vi "Primitives.vi"(1 "Angle to Target":i32, 5 "Primitive":string, 8 "Distance to Target":i32) -> (0 "Port Speed":i32, 6 "Starboard Speed":i32)   [LabVIEW 2012]
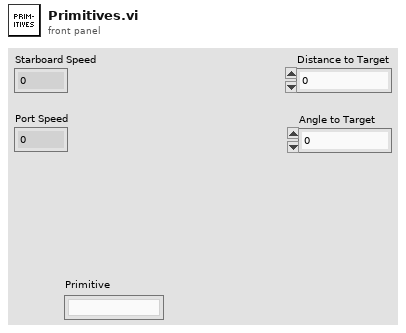
[diagram p1: front panel]
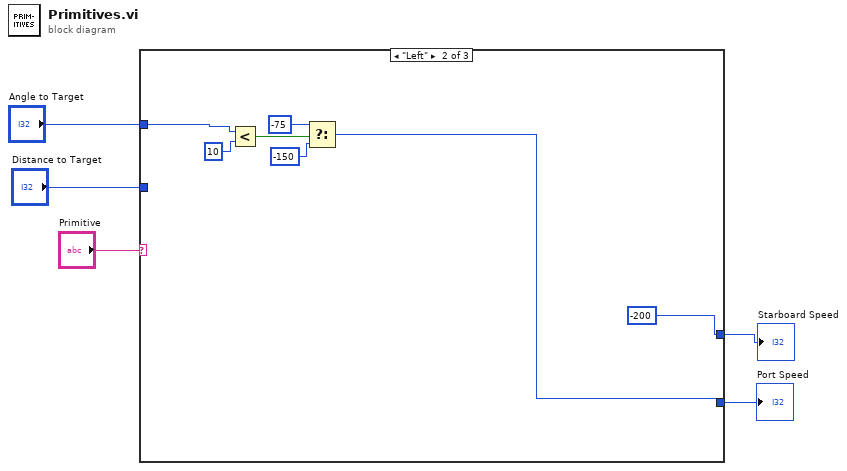
[diagram p0: block diagram]
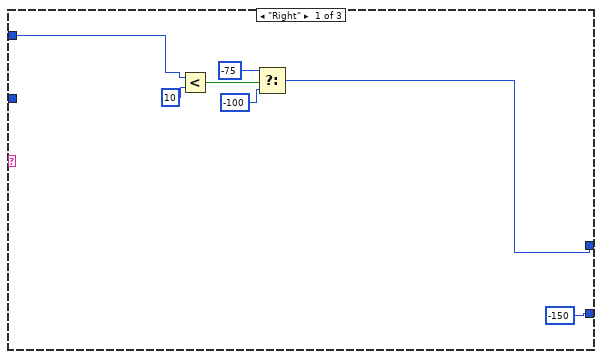
[diagram p2: hidden frame]
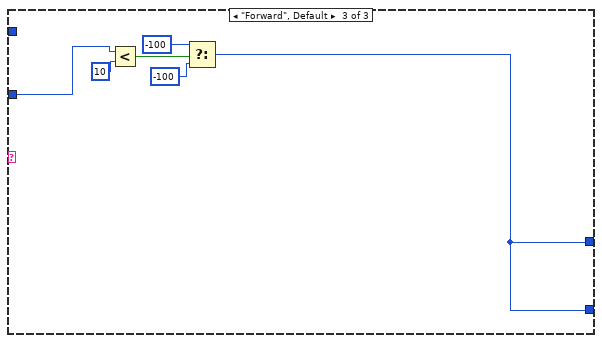
[diagram p3: hidden frame]
diagram:
  n1 = case shown="\"Left\"" "Primitive" {
    tunnel: [w7 -200 w22] -> w4
    tunnel: [-150 w14 w22] -> w3
    tunnel: "Angle to Target" -> [w8 w15 _]
    tunnel: "Distance to Target" -> [_ _ w25]
    frame "Right" {
      n2 = Less?(x=w8, y=10) -> (x < y?=w11:bool)
      n3 = Select(t=-75, s=w11, f=-100) -> (s? t:f=w7:i32)
    }
    frame "Left" {
      n4 = Less?(x=w15, y=10) -> (x < y?=w18:bool)
      n5 = Select(t=-75, s=w18, f=-150) -> (s? t:f=w14:i32)
    }
    frame "Forward", Default {
      n6 = Less?(x=w25, y=10) -> (x < y?=w23:bool)
      n7 = Select(t=-100, s=w23, f=-100) -> (s? t:f=w22:i32)
    }
  }
  "Starboard Speed" <- w4
  "Port Speed" <- w3
